vi "UI.Stream.Disable.vi"(8 "error in (no error)":errorcluster, 11 "State Variables in":T1) -> (0 "error out":errorcluster)   [LabVIEW 2023, in "Protection and Counter Workspace Shared.lvlib"]
uses:
  Protection and Counter Workspace Shared.lvlib
  Types/Workspace.State.ctl
  Types/UI.Refs.ctl
  SubModules/CAN-Streaming-Support/Source/Addon/Addon Shared/Types/Type Filter.ctl
  <vilib>/NI VeriStand/Display Template Support/DisplayTemplateSupport.llb/enum_Display Template Handler Minimal To Workspace.ctl
  Types/Workspace.SavedState.ctl
  NationalInstruments.VeriStand.SystemStorage
  <vilib>/NI VeriStand/Execution/Workspace/WorkspaceAPI.ctl
  NationalInstruments.VeriStand.ClientAPI
  <vilib>/NI VeriStand/Display Template Support/DisplayTemplateSupport.llb/enum_Display Template Handler Minimal To Widget Msg.ctl
  <vilib>/NI VeriStand/Execution/Workspace/SystemStateRegEventRef.ctl
  <vilib>/NI VeriStand/Execution/Workspace/Target State Info.ctl
  <vilib>/NI VeriStand/Execution/Workspace/Target State.ctl
  <vilib>/NI VeriStand/Execution/Workspace/SystemStateEventRef.ctl
  SubModules/CAN-Streaming-Support/Source/UIs/Workspace Shared/Types/Host Stream Queue Refs.ctl
  SubModules/CAN-Streaming-Support/Source/UIs/Workspace Shared/Types/Host Stream Queue Type.ctl
  SubModules/CAN-Streaming-Support/Source/UIs/Workspace Shared/Types/Host Stream Queue Command.ctl
  <vilib>/xnet/xnet.llb/XNET Frame CAN.ctl
  <vilib>/xnet/xnet.llb/XNET Frame Type CAN.ctl
  <vilib>/Utility/miscctls.llb/LVRowAndColumnUnsignedTypeDef.ctl
  <vilib>/NI VeriStand/Execution/Workspace/NI_VS Workspace ExecutionAPI.lvlib
  SubModules/CAN-Streaming-Support/Source/UIs/Workspace Shared/CAN Stream Support Workspace Shared.lvlib
  SubModules/CAN-Streaming-Support/Source/Addon/Addon Shared/CAN Stream Support Shared.lvlib
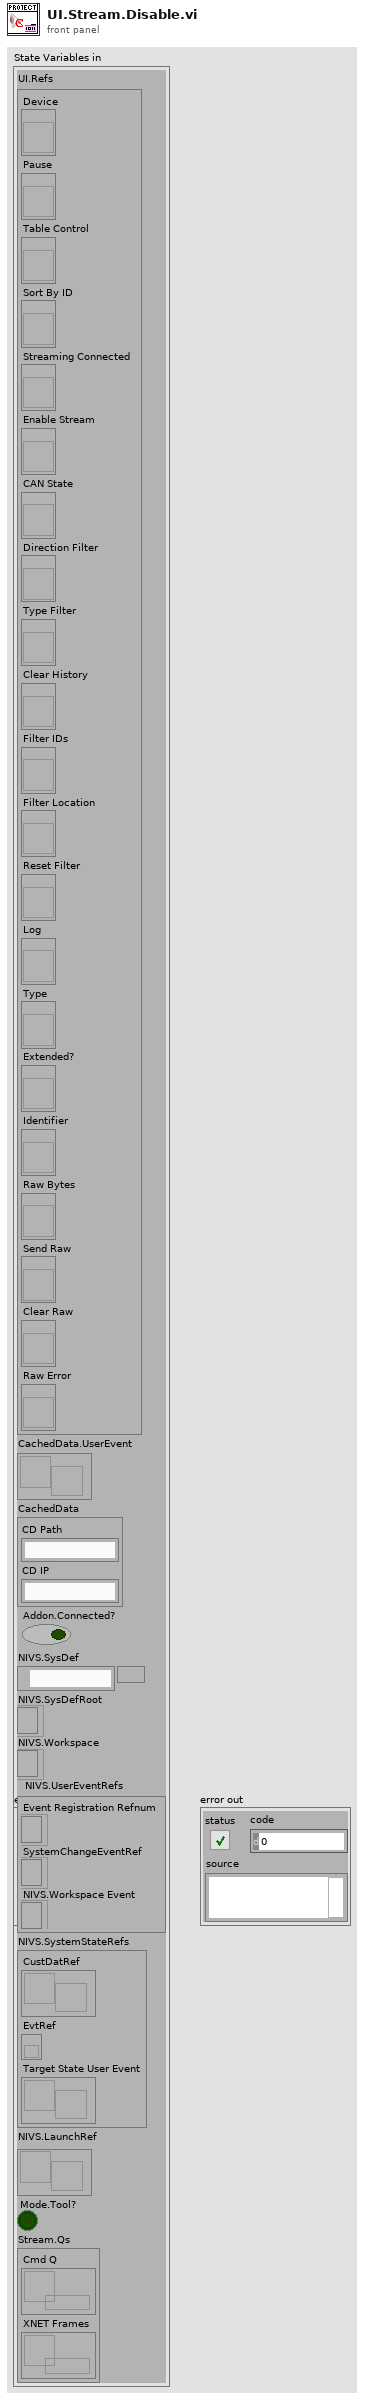
[diagram p1: front panel]
types:
  T1 = typedef "Protection and Counter Workspace Shared.lvlib/Workspace.State.ctl" = cluster{"UI.Refs":T2, "CachedData.UserEvent":refnum<user-event>, "CachedData":T3, "Addon.Connected?":bool, "NIVS.SysDef":path, "NIVS.SysDefRoot":refnum<k24>, "NIVS.Workspace":T4, "NIVS.UserEventRefs":cluster{"Event Registration Refnum":refnum<event-registration>, "SystemChangeEventRef":T5, "NIVS.Workspace Event":refnum<event-registration>}, "NIVS.SystemStateRefs":T6, "NIVS.LaunchRef":refnum<user-event>, "Mode.Tool?":bool, "Stream.Qs":T7}
  T2 = typedef "Protection and Counter Workspace Shared.lvlib/UI.Refs.ctl" = cluster{"Device":refnum<vi>, "Pause":refnum<vi>, "Table Control":refnum<vi>, "Sort By ID":refnum<vi>, "Streaming Connected":refnum<vi>, "Enable Stream":refnum<vi>, "CAN State":refnum<vi>, "Direction Filter":refnum<vi>, "Type Filter":refnum<vi>, "Clear History":refnum<vi>, "Filter IDs":refnum<vi>, "Filter Location":refnum<vi>, "Reset Filter":refnum<vi>, "Log":refnum<vi>, "Type":refnum<vi>, "Extended?":refnum<vi>, "Identifier":refnum<vi>, "Raw Bytes":refnum<vi>, "Send Raw":refnum<vi>, "Clear Raw":refnum<vi>, "Raw Error":refnum<vi>}
  T3 = typedef "Protection and Counter Workspace Shared.lvlib/Workspace.SavedState.ctl" = cluster{"CD Path":string, "CD IP":string}
  T4 = typedef "NI_VS Workspace ExecutionAPI.lvlib/WorkspaceAPI.ctl" = refnum<k24>
  T5 = typedef "NI_VS Workspace ExecutionAPI.lvlib/SystemStateRegEventRef.ctl" = refnum<event-registration>
  T6 = typedef "NI_VS Workspace ExecutionAPI.lvlib/SystemStateEventRef.ctl" = cluster{"CustDatRef":refnum<user-event>, "EvtRef":refnum<k27>, "Target State User Event":refnum<user-event>}
  T7 = typedef "CAN Stream Support Workspace Shared.lvlib/Host Stream Queue Refs.ctl" = cluster{"Cmd Q":refnum<queue>, "XNET Frames":refnum<queue>}
  T8 = typedef "LVRowAndColumnUnsignedTypeDef.ctl" = cluster{"Row":u32, "Column":u32}
  T9 = enum8{"Enabled", "Disabled", "Disabled and Grayed Out"}
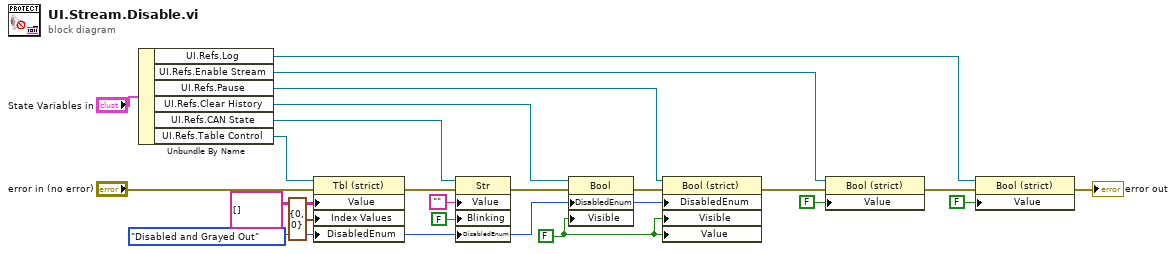
[diagram p0: block diagram]
diagram:
  w9 = FALSE ("Value")
  w10 = T9."Disabled and Grayed Out" ("Disabled")
  n1 = Unbundle By Name("State Variables in") -> ("UI.Refs.Log"=w2:refnum<vi>, "UI.Refs.Enable Stream"=w7:refnum<vi>, "UI.Refs.Pause"=w11:refnum<vi>, "UI.Refs.Clear History"=w14:refnum<vi>, "UI.Refs.CAN State"=w19:refnum<vi>, "UI.Refs.Table Control"=w21:refnum<vi>)
  n2 = property class="Tbl (strict)"(reference=w21, error in="error in (no error)", "Value"=string[][] [], "Index Values"=T8 {"Row"=0, "Column"=0}, "DisabledEnum"=w10) -> (error out=w15:errorcluster)  [unwired: 1 out]
  n3 = property class="Str"(reference=w19, error in=w15, "Value"="", "Blinking"=FALSE, "DisabledEnum"=w10) -> (error out=w13:errorcluster)  [unwired: 1 out]
  n4 = property class="Bool"(reference=w14, error in=w13, "DisabledEnum"=w10, "Visible"=w9) -> (error out=w12:errorcluster)  [unwired: 1 out]
  n5 = property class="Bool (strict)"(reference=w11, error in=w12, "DisabledEnum"=w10, "Visible"=w9, "Value"=w9) -> (error out=w6:errorcluster)  [unwired: 1 out]
  n6 = property class="Bool (strict)"(reference=w7, error in=w6, "Value"=FALSE ("Visible")) -> (error out=w4:errorcluster)  [unwired: 1 out]
  n7 = property class="Bool (strict)"(reference=w2, error in=w4, "Value"=FALSE ("Visible")) -> (error out=→"error out":errorcluster)  [unwired: 1 out]
